vi "Graph_Flow_testing.vi"(0 "Cluster":T2, 2 "START\nTHRESHOLD\nTRIGGER\nindex 2":i32, 3 "Filtered \nSize Length":i32, 5 "error in":errorcluster, 6 "CSV file path":path) -> (14 "MIN_MAX_FLOW":bool, 15 "Filter Graph Flow":cluster{timestamp[], ext[]}(graph), 16 "MAX-MIN_Flow":cluster{"MIN":dbl, "MAX":dbl, "ACTUAL":dbl}, 19 "error out":errorcluster)   [LabVIEW 2017]
uses:
  <vilib>/Utility/file.llb/Read Delimited Spreadsheet (string).vi
panel:
  out "Flow":T1
  out "input filter array":ext[](array[numeric])
  out "Normal Graph":cluster{timestamp[], ext[]}(graph)
  out "time stamp":timestamp[](array[timestamp])
  out "input unfilter array":ext[](array[numeric])
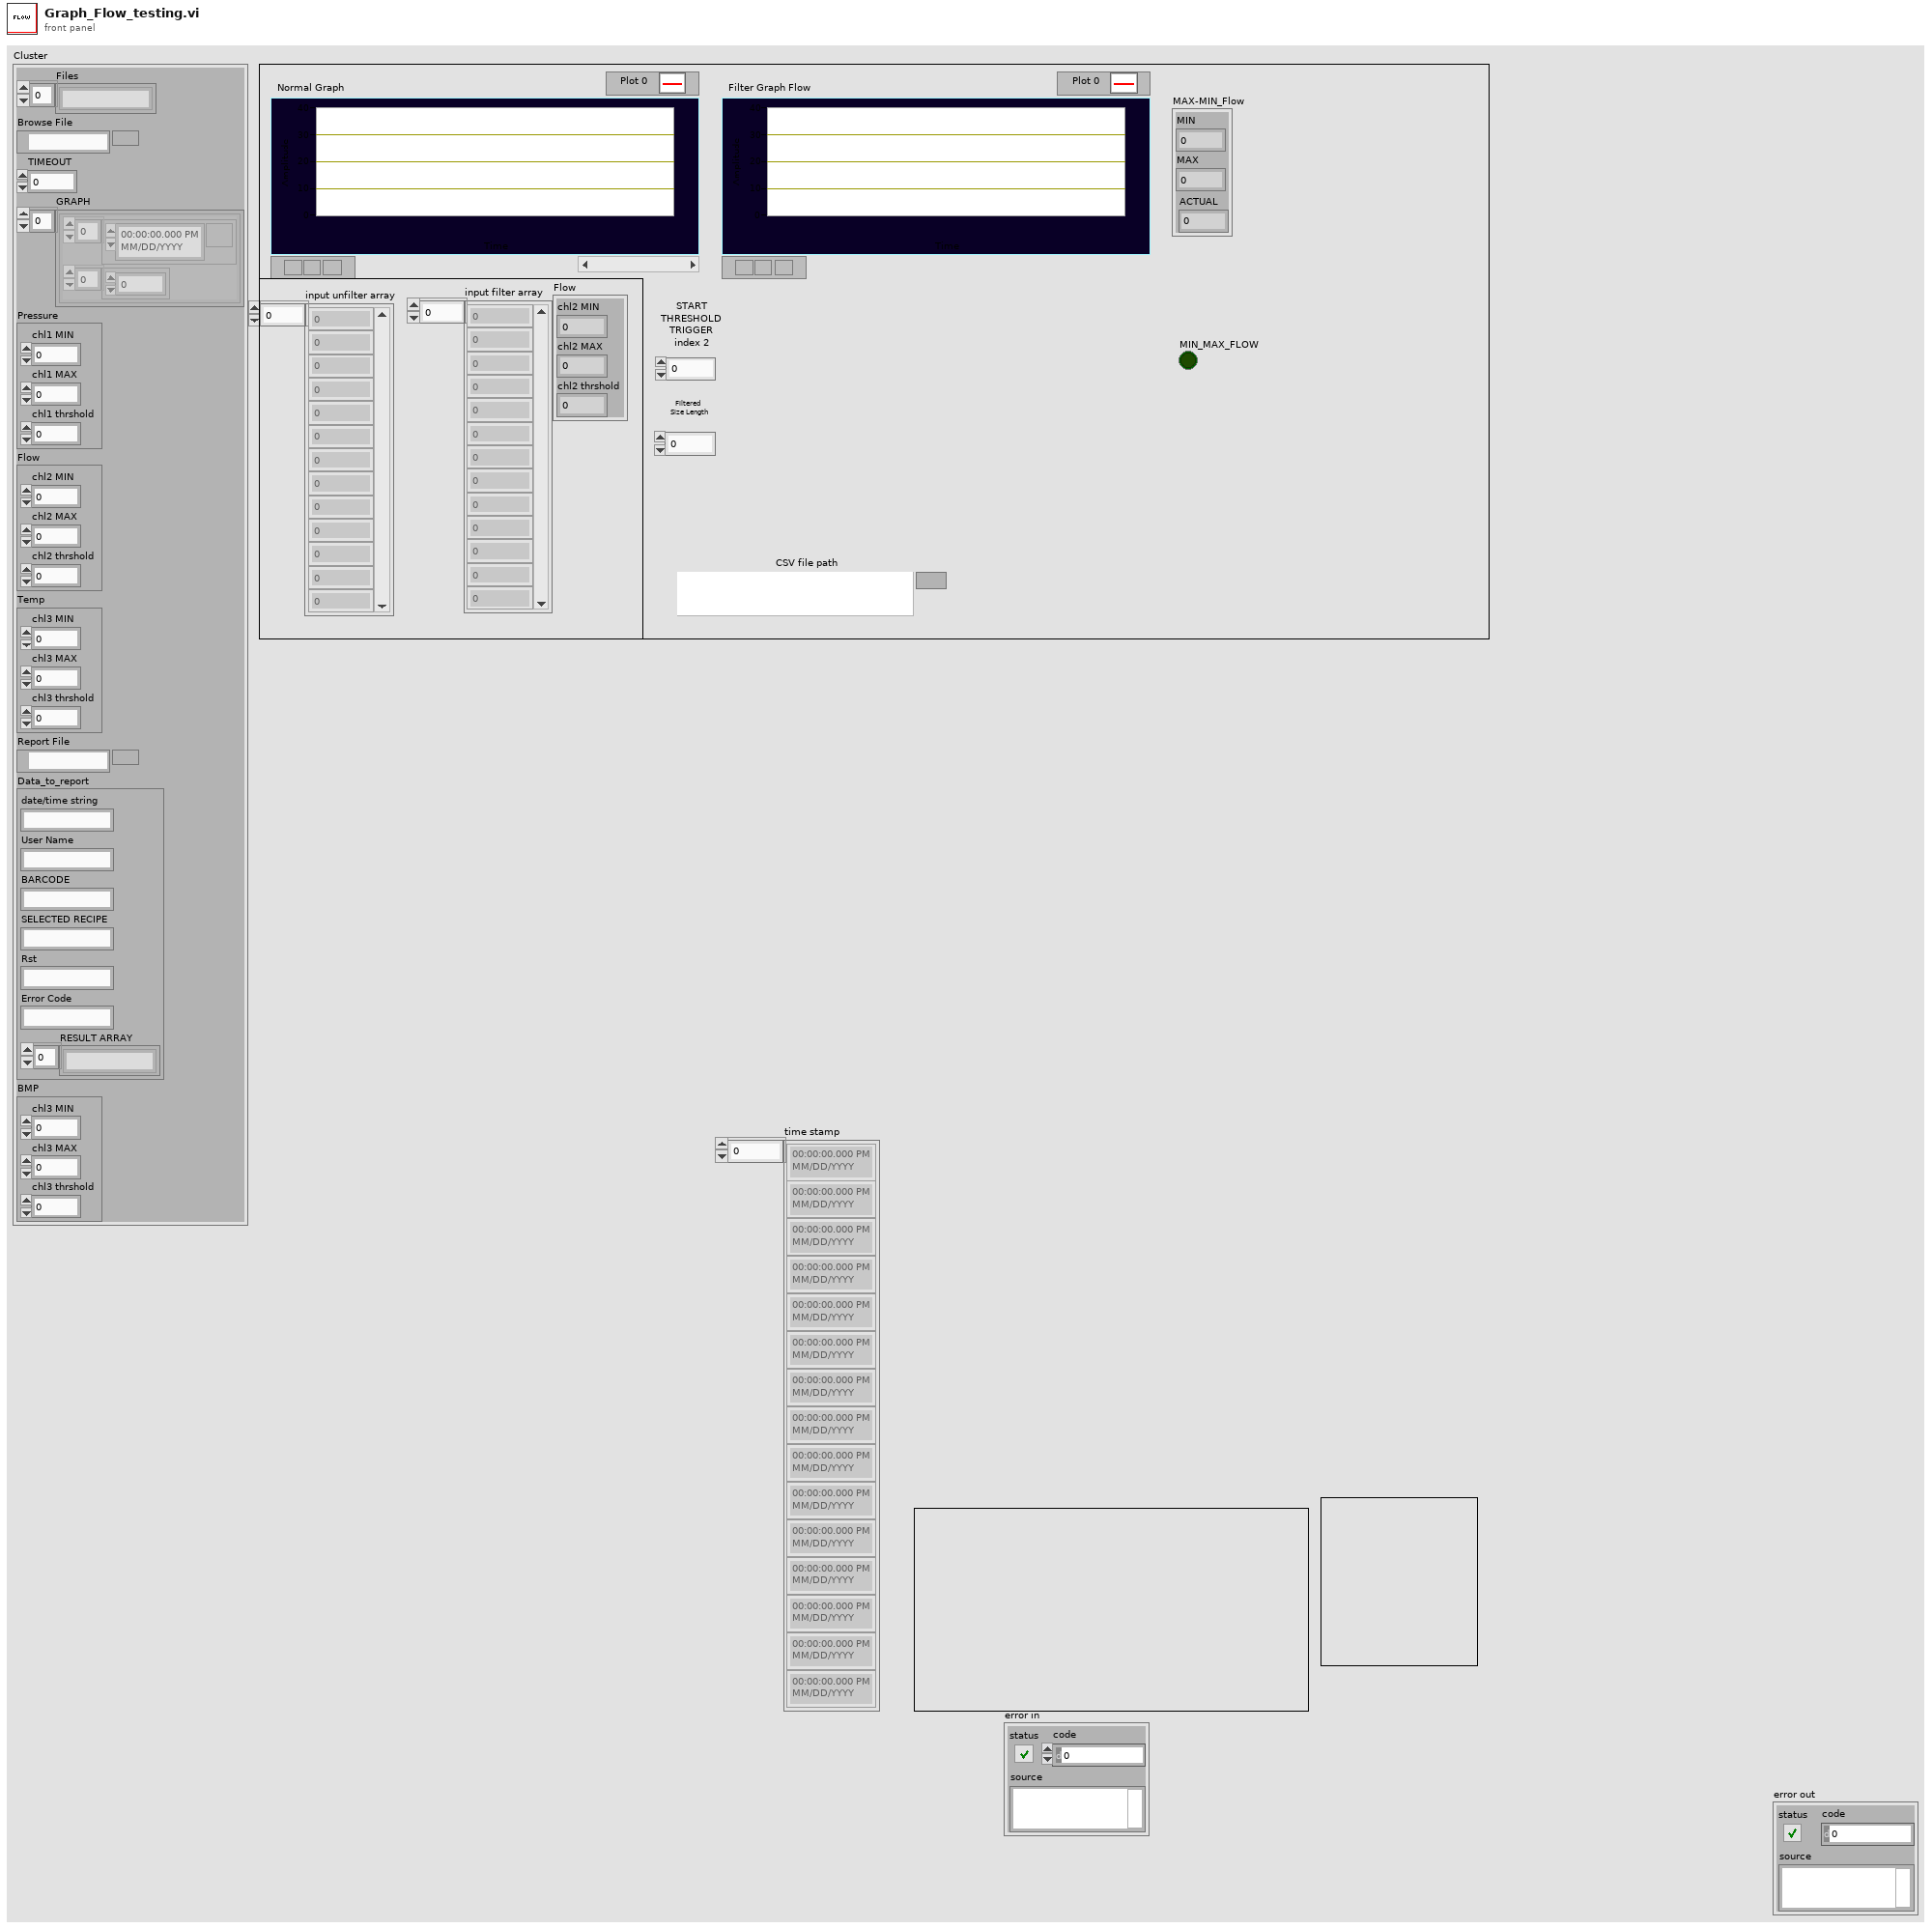
[diagram p1: front panel]
types:
  T1 = cluster{"chl2 MIN":dbl, "chl2 MAX":dbl, "chl2 thrshold":dbl}
  T2 = cluster{"Files":string[], "Browse File":path, "TIMEOUT":i32, "GRAPH":cluster{timestamp[], ext[]}[], "Pressure":cluster{"chl1 MIN":dbl, "chl1 MAX":dbl, "chl1 thrshold":dbl}, "Flow":cluster{"chl2 MIN":dbl, "chl2 MAX":dbl, "chl2 thrshold":dbl}, "Temp":cluster{"chl3 MIN":dbl, "chl3 MAX":dbl, "chl3 thrshold":dbl}, "Report File":path, "Data_to_report":cluster{"date/time string":string, "User Name":string, "BARCODE":string, "SELECTED RECIPE":string, "Rst":string, "Error Code":string, "RESULT ARRAY":string[]}, "BMP":cluster{"chl3 MIN":dbl, "chl3 MAX":dbl, "chl3 thrshold":dbl}}
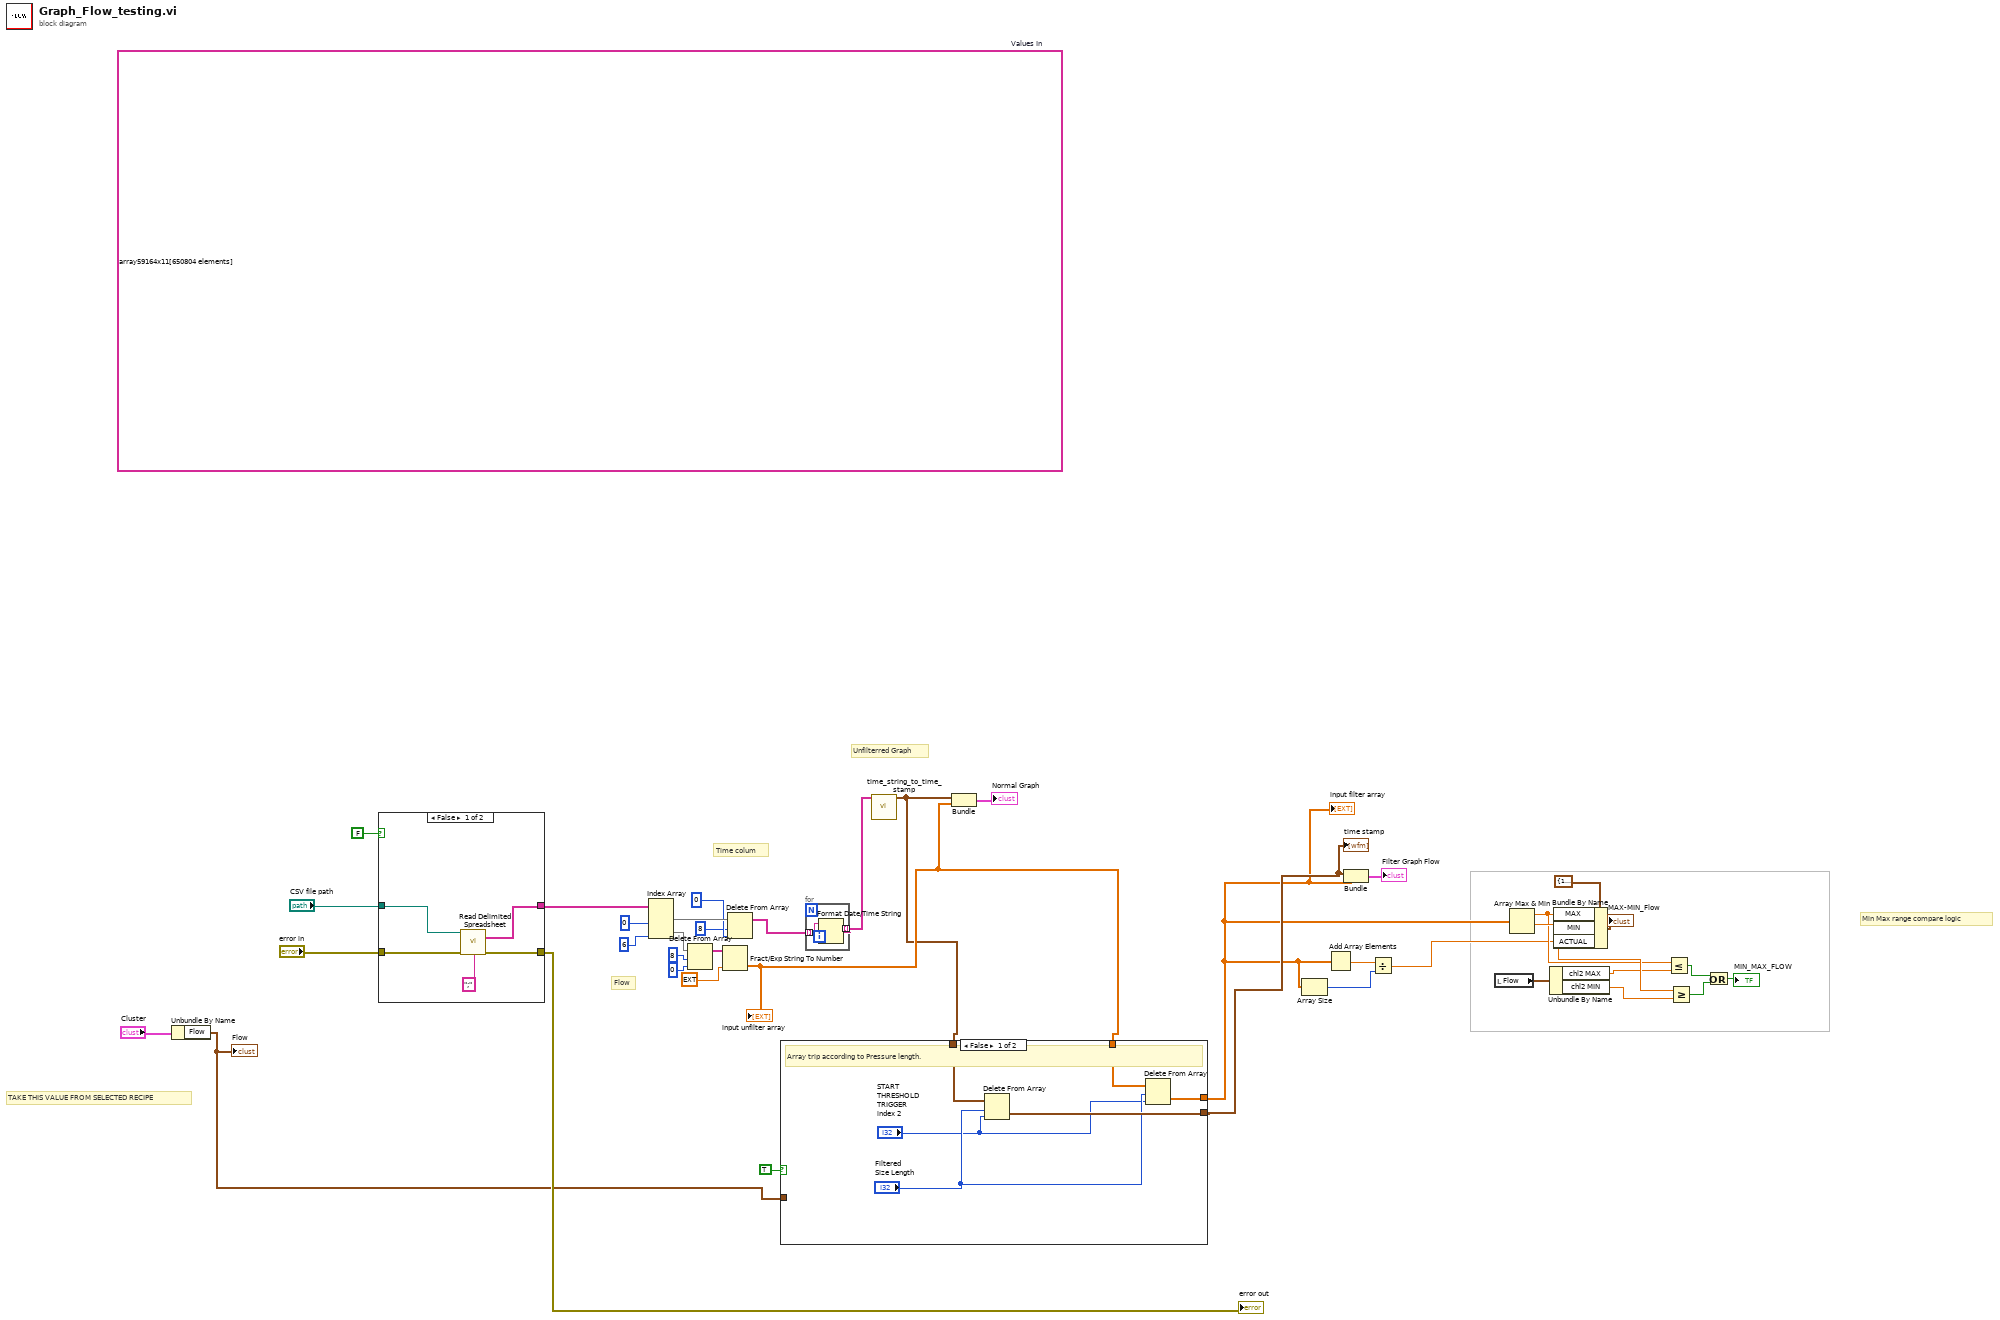
[diagram p0: block diagram]
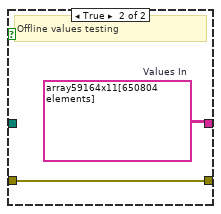
[diagram p3: hidden frame]
diagram:
  (unwired) string[][] array59164x11[650804 elements]  # Values In
  # "Flow"
  # "Min Max range compare logic"
  # "Unfilterred Graph"
  # "Time colum"
  # "TAKE THIS VALUE FROM SELECTED RECIPE"
  n1 = Unbundle By Name("Cluster") -> ("Flow"=w1:T1)
  "Flow" <- w1
  n2 = case shown="False" FALSE {
    tunnel: [w43 w46] -> w34
    tunnel: "CSV file path" -> [w42 _]
    tunnel: [w41 w45] -> w27
    tunnel: "error in" -> [w40 w45]
    frame False {
      n3 = call-poly <vilib>:"Read Delimited Spreadsheet.vi"("file path (dialog if empty)"=w42, "error in (no error)"=w40, "delimiter (\\t)"=";" ("delimiter (\\t)")) -> ("all rows"=w43:string[][], "error out"=w41:errorcluster)  [unwired: 7 in, 4 out]
    }
    frame True {
      w46 = string[][] array59164x11[650804 elements]  # Values In
      # "Offline values testing"
    }
  }
  "error out" <- w27
  n4 = Index Array(array=w34, index (col) #1=0 ("index (row)"), index (col) #2=6 ("index (row)")) -> (element #1=w39:string[], element #2=w35:string[])  [unwired: 2 in]
  n5 = Delete From Array(array=w35, length=8 ("index (row)"), index=0 ("index (row)")) -> (array with subset deleted=w30:string[])  [unwired: 1 out]
  n6 = Fract/Exp String To Number(string=w30, default (0 dbl)=ext 0.0 ("String")) -> (number=w15:ext[])  [unwired: 2 in, 1 out]
  "input unfilter array" <- w15
  n7 = Delete From Array(array=w39, length=8 ("index (row)"), index=0 ("index (row)")) -> (array with subset deleted=w21:string[])  [unwired: 1 out]
  n8 = for {
    tunnel: w21 -> [w48] mode=indexing
    tunnel: [w47] -> w16 mode=indexing
    n9 = Format Date/Time String(time format string (%c)=w48) -> (date/time string=w47:string)  [unwired: 2 in]
  }
  n10 = call "time_string_to_time_stamp.vi"("Array in"=w16) -> ("Array out"=w13:timestamp[])  [unwired: 10 in]
  n11 = case shown="False" TRUE {
    tunnel: w1 -> [_ _]
    tunnel: w13 -> [w54 w55]
    tunnel: [w53 w55] -> w14
    tunnel: w15 -> [w50 w56]
    tunnel: [w49 w56] -> w6
    frame False {
      # "Array trip according to Pressure length."
      n12 = Delete From Array(array=w54, length="Filtered \nSize Length", index="START\nTHRESHOLD\nTRIGGER\nindex 2") -> (deleted portion=w53:timestamp[])  [unwired: 1 out]
      n13 = Delete From Array(array=w50, length="Filtered \nSize Length", index="START\nTHRESHOLD\nTRIGGER\nindex 2") -> (deleted portion=w49:ext[])  [unwired: 1 out]
    }
    frame True {
      # "Direct value from array of temp"
    }
  }
  "time stamp" <- w14
  "input filter array" <- w6
  n14 = Bundle("Array out"=w13, w15) -> (→"Normal Graph":cluster{"Array out":timestamp[], ext[]})  [unwired: 1 in]
  n15 = Array Size(array=w6) -> (size(s)=w4:i32)
  n16 = Add Array Elements(numeric array=w6) -> (sum=w5:ext)
  n17 = Bundle("Array out"=w14, w6) -> (→"Filter Graph Flow":cluster{"Array out":timestamp[], ext[]})  [unwired: 1 in]
  n18 = Divide(x=w5, y=w4) -> (x/y=w3:ext)
  n19 = local read "Flow"() -> (w20:T1)
  n20 = Array Max & Min(array=w6) -> (max value=w8:ext, min value=w12:ext)  [unwired: 2 out]
  n21 = Unbundle By Name(w20) -> ("chl2 MAX"=w7:dbl, "chl2 MIN"=w11:dbl)
  n22 = Bundle By Name(cluster=cluster{"MIN":dbl, "MAX":dbl, "ACTUAL":dbl} {"MIN"=110.0, "MAX"=130.0, "ACTUAL"=0.0} ("CHL 2"), "MAX"=w8, "MIN"=w12, "ACTUAL"=w3) -> (→"MAX-MIN_Flow":cluster{"MIN":dbl, "MAX":dbl, "ACTUAL":dbl})
  n23 = Less Or Equal?(x=w8, y=w7) -> (x <= y?=w9:bool)
  n24 = Greater Or Equal?(x=w12, y=w11) -> (x >= y?=w10:bool)
  n25 = Or(x=w9, y=w10) -> (x .or. y?=→"MIN_MAX_FLOW":bool)
